vi "greater Unit Test.vi"(7 "x+y":dbl, 8 "entrée d'erreur (pas d'erreur)":errorcluster, 9 "Label":string, 10 "String 2":string, 11 "String":string) -> (0 "sortie d'erreur":errorcluster)   [LabVIEW 2021]
uses:
  <vilib>/addons/_JKI Toolkits/Caraya/classes/Properties.Assert/Properties.Assert.lvclass
  C:/Program Files (x86)/National Instruments/LabVIEW 2021/vi.lib/addons/_JKI Toolkits/Caraya/classes/Properties/Properties.lvclass
  <vilib>/addons/_JKI Toolkits/Caraya/classes/Assert/Assert Greater Or Equal_Variant.vi
  <vilib>/addons/_JKI Toolkits/Caraya/classes/Assert/Assert.lvclass
  <vilib>/addons/_JKI Toolkits/Caraya/classes/Properties/Properties.lvclass
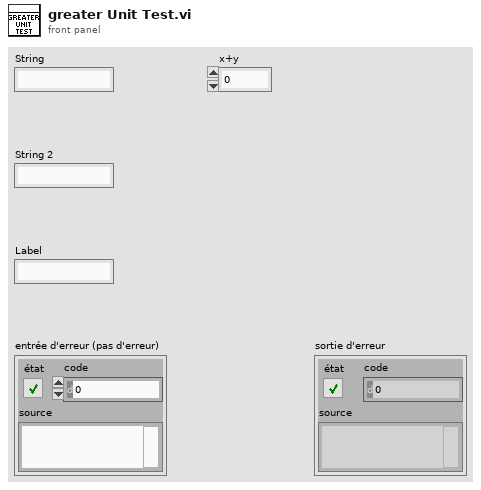
[diagram p1: front panel]
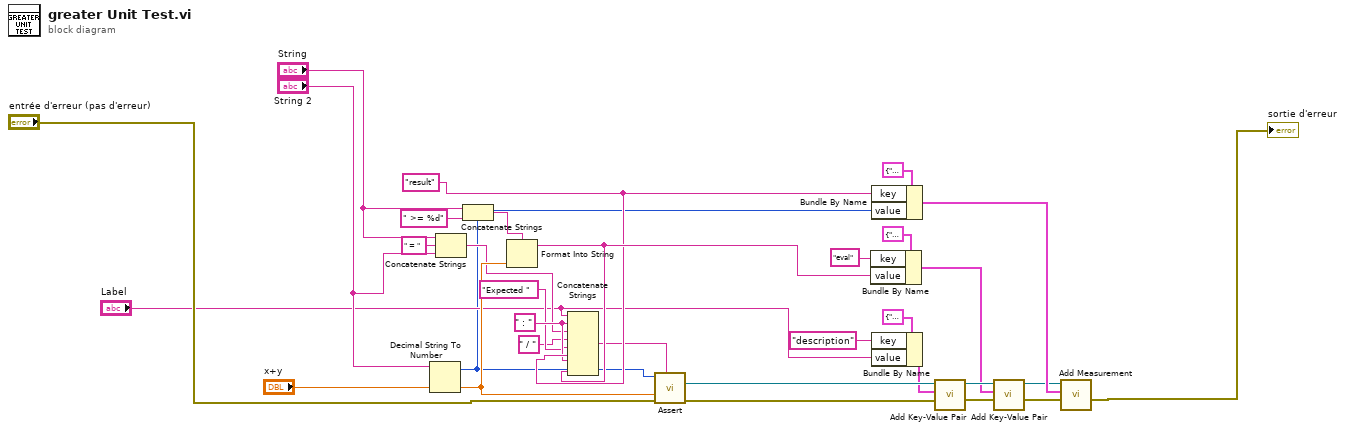
[diagram p0: block diagram]
diagram:
  w23 = " : " ("chaîne")
  w24 = "result"
  n1 = Decimal String To Number(string="String 2") -> (offset past number=w15:i32)  [unwired: 2 in, 1 out]
  n2 = Concatenate Strings("String", " = " ("chaîne"), "String 2") -> (w21:string)
  n3 = Concatenate Strings("String", " >= %d" ("chaîne")) -> (w28:string)
  n4 = Format Into String(format string=w28, "x+y") -> (resulting string=w29:string)  [unwired: 2 in, 1 out]
  n5 = Concatenate Strings("Label", w23, w21, " / " ("chaîne"), "Expected " ("chaîne"), w24, w23, w29) -> (w20:string)
  n6 = call-poly <vilib>:"Assert.vi"("Label"=w20, "error in (no error)"="entrée d'erreur (pas d'erreur)", "Y"="x+y", "X"=w15) -> ("error out"=w13:errorcluster, "Properties.Assert"=w14:refnum<class "Properties.Assert.lvclass">)  [unwired: 6 in]
  n7 = Bundle By Name(cluster=cluster{"key":string, "value":variant} {"key"="", "value"=variant} ("entry"), "key"="eval", "value"=w29) -> (w2:cluster{"key":string, "value":variant})
  n8 = Bundle By Name(cluster=cluster{"key":string, "value":variant} {"key"="", "value"=variant} ("entry"), "key"=w24, "value"=w15) -> (w8:cluster{"key":string, "value":variant})
  n9 = Bundle By Name(cluster=cluster{"key":string, "value":variant} {"key"="", "value"=variant} ("entry"), "key"="description", "value"="Label") -> (w11:cluster{"key":string, "value":variant})
  n10 = call <vilib>:"Add Key-Value Pair.vi"("error in (no error)"=w13, "entry"=w11, "Properties in"=w14) -> ("error out"=w7:errorcluster, "Properties out"=w5:refnum<class "Properties.Assert.lvclass">)  [unwired: 7 in]
  n11 = call <vilib>:"Add Key-Value Pair.vi"("error in (no error)"=w7, "entry"=w2, "Properties in"=w5) -> ("error out"=w6:errorcluster, "Properties out"=w4:refnum<class "Properties.Assert.lvclass">)  [unwired: 7 in]
  n12 = call <vilib>:"Add Measurement.vi"("error in (no error)"=w6, "entry"=w8, "Properties"=w4) -> ("error out"=→"sortie d'erreur":errorcluster)  [unwired: 7 in, 1 out]
